vi "FIFO IN.vi"(8 "error in (no error)":errorcluster, 11 "Engine Run-Time Data Cluster In":T1 {"Compiled Data"."Corruption Info DUT_Network"."Frame Infos Array"."CRC Index" min=-7 max=7; "Compiled Data"."Corruption Info DUT_Network"."Frame Infos Array"."DLC Length  Corruption Index" min=-8 max=8; "Compiled Data"."Corruption Info Network_DUT"."Frame Infos Array"."CRC Index" min=-7 max=7; "Compiled Data"."Corruption Info Network_DUT"."Frame Infos Array"."DLC Length  Corruption Index" min=-8 max=8; "Specified Channel Ref List Out" format="%.0x"; "Specified Channel Ref List In" format="%.0x"}) -> (0 "error out":errorcluster, 3 "Engine Run-Time Data Cluster Out":T1 {"Compiled Data"."Corruption Info DUT_Network"."Frame Infos Array"."CRC Index" min=-7 max=7; "Compiled Data"."Corruption Info DUT_Network"."Frame Infos Array"."DLC Length  Corruption Index" min=-8 max=8; "Compiled Data"."Corruption Info Network_DUT"."Frame Infos Array"."CRC Index" min=-7 max=7; "Compiled Data"."Corruption Info Network_DUT"."Frame Infos Array"."DLC Length  Corruption Index" min=-8 max=8; "Specified Channel Ref List Out" format="%.0x"; "Specified Channel Ref List In" format="%.0x"})   [LabVIEW 2018, in "CAN Gateway Engine.lvlib"]
uses:
  CAN Gateway Engine.lvlib
  Shared/CTLs/Runtime engine Data.ctl
  <vilib>/NI Veristand/Custom Device API/Custom Device Engine Event Ref.ctl
  <vilib>/NI Veristand/Custom Device API/Custom Device Item Ref.ctl
  Shared/CTLs/Compiled Data.ctl
  Shared/CTLs/Corruption Info.ctl
  Shared/CTLs/Frame.ctl
  Shared/CTLs/Signal_Data_Trigger.ctl
  <vilib>/NI Veristand/Custom Device API/Custom Device API.lvlib
  Shared/CAN Gateway Shared.lvlib
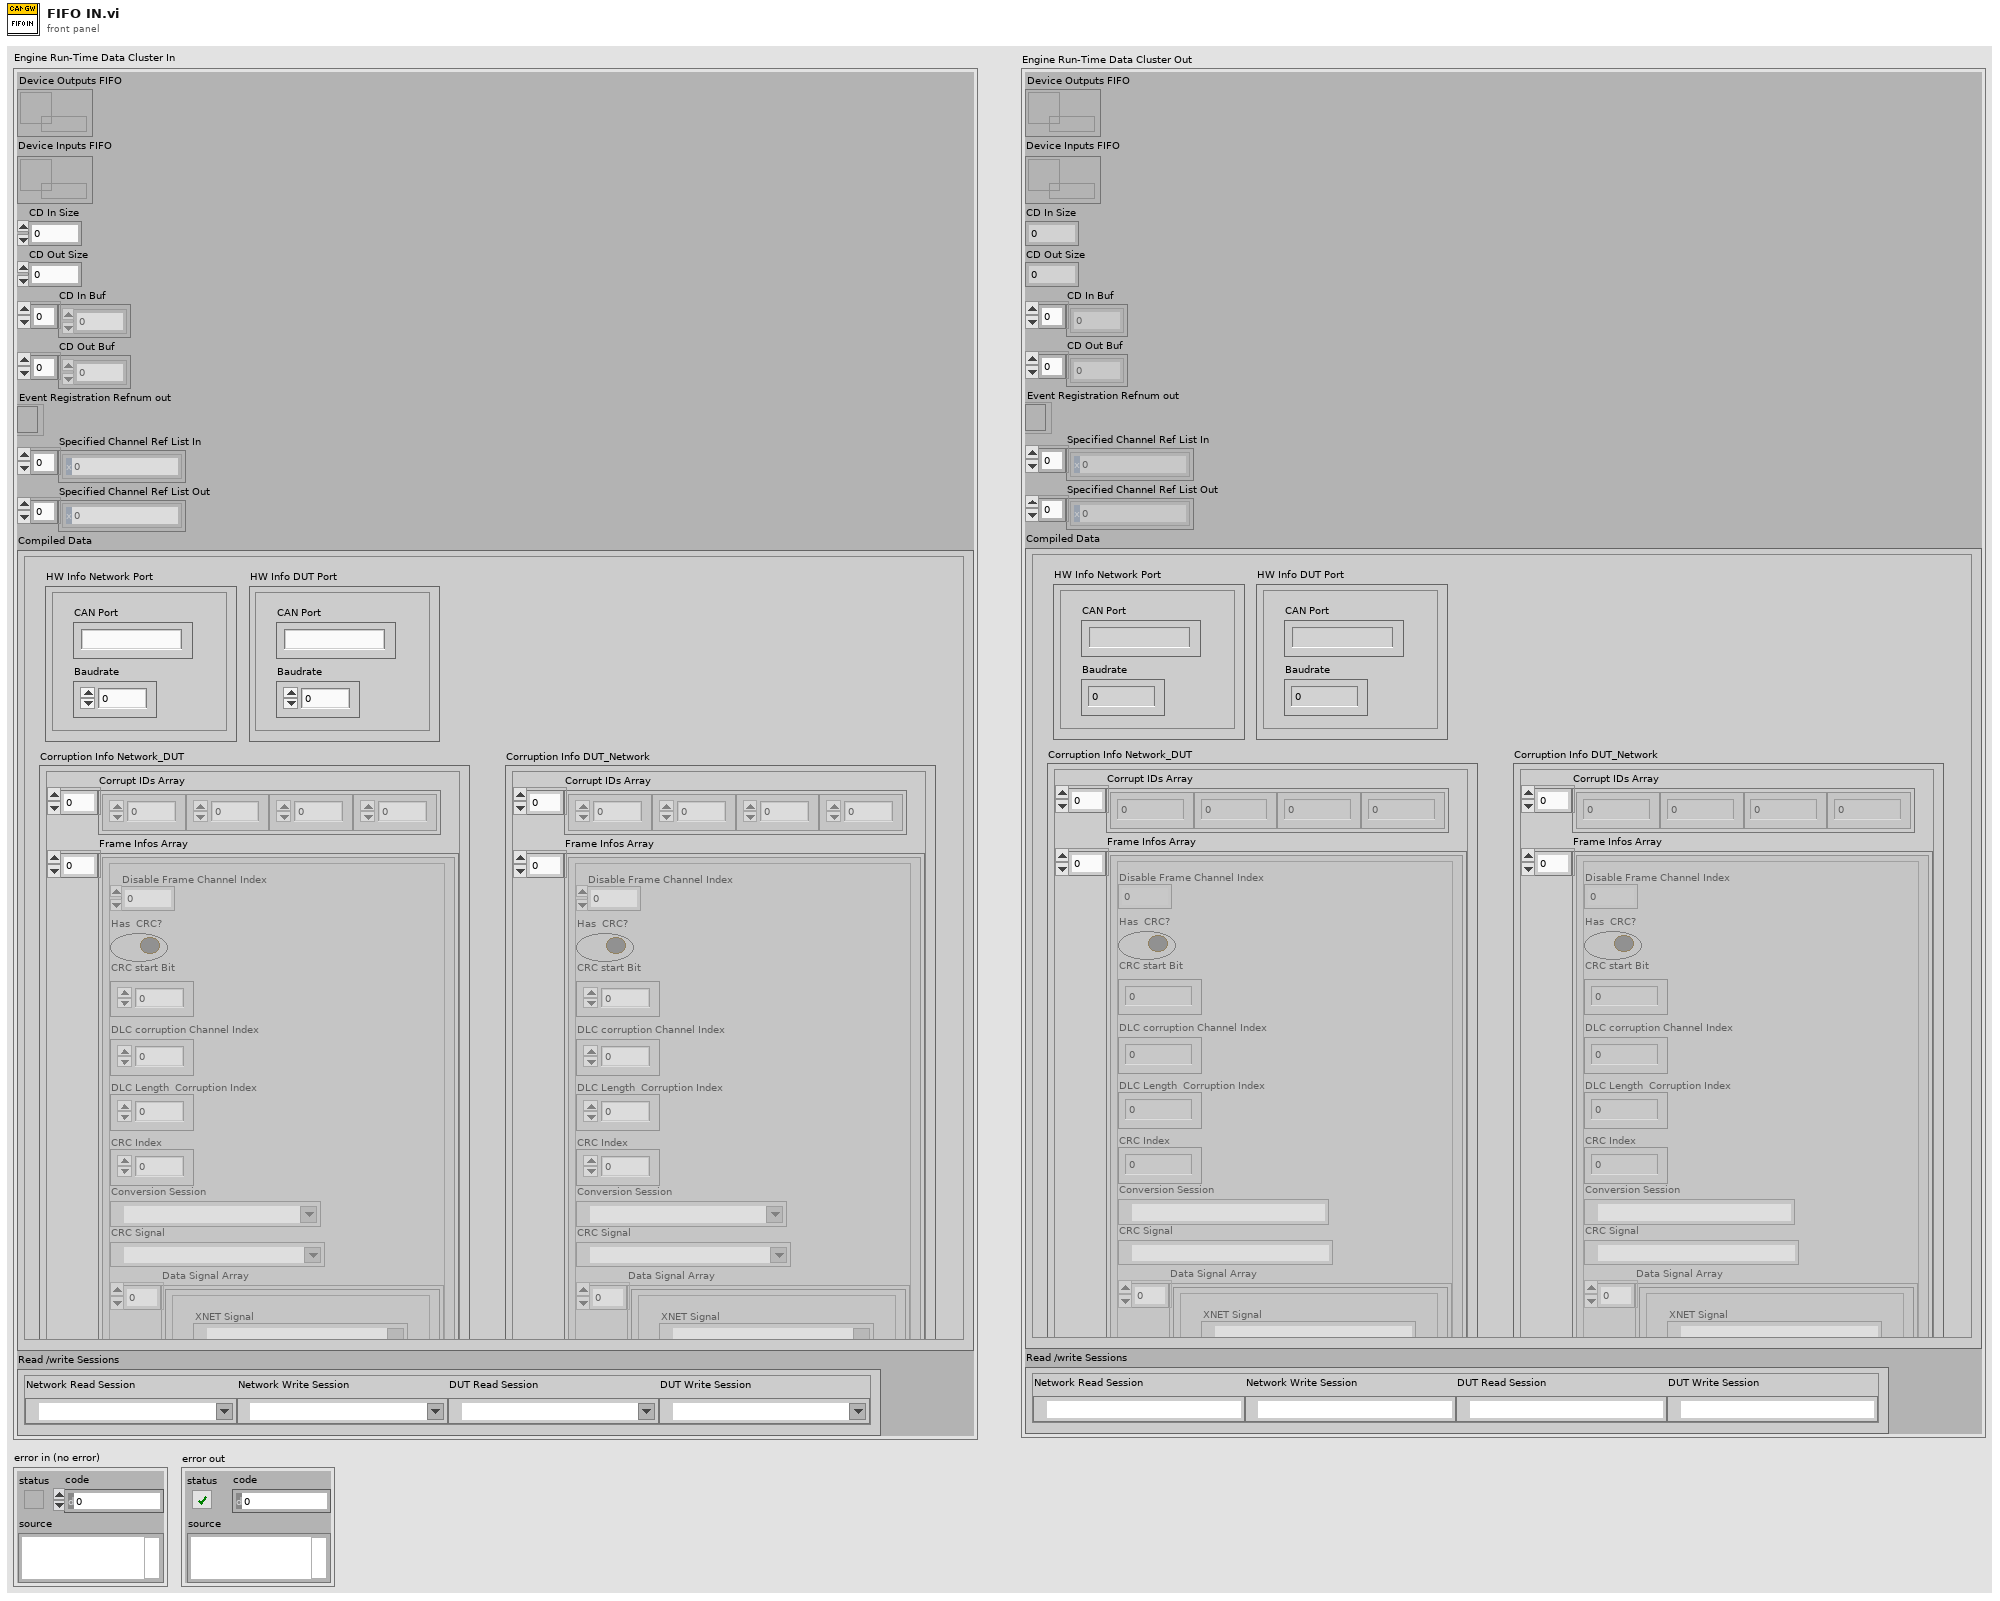
[diagram p1: front panel]
types:
  T1 = typedef "CAN Gateway Engine.lvlib/Runtime engine Data.ctl" = cluster{"Device Outputs FIFO":refnum<k33>, "Device Inputs FIFO":refnum<k33>, "CD In Size":i32, "CD Out Size":i32, "CD In Buf":dbl[], "CD Out Buf":dbl[], "Event Registration Refnum out":T2, "Specified Channel Ref List In":T3[], "Specified Channel Ref List Out":T3[], "Compiled Data":T4, "Read /write Sessions":cluster{"Network Read Session":refnum<k21>, "Network Write Session":refnum<k21>, "DUT Read Session":refnum<k21>, "DUT Write Session":refnum<k21>}}
  T2 = typedef "Custom Device API.lvlib/Custom Device Engine Event Ref.ctl" = refnum<event-registration>
  T3 = typedef "Custom Device API.lvlib/Custom Device Item Ref.ctl" = u64
  T4 = typedef "CAN Gateway Shared.lvlib/Compiled Data.ctl" = cluster{"HW Info Network Port":cluster{"CAN Port":string, "Baudrate":u64}, "HW Info DUT Port":cluster{"CAN Port":string, "Baudrate":u64}, "Corruption Info Network_DUT":T5, "Corruption Info DUT_Network":T5}
  T5 = typedef "CAN Gateway Shared.lvlib/Corruption Info.ctl" = cluster{"Corrupt IDs Array":u32[], "Frame Infos Array":T6[]}
  T6 = typedef "CAN Gateway Shared.lvlib/Frame.ctl" = cluster{"Disable Frame Channel Index":i32, "Has  CRC?":bool, "CRC start Bit":u32, "DLC corruption Channel Index":i32, "DLC Length  Corruption Index":i32, "CRC Index":i32, "Conversion Session":refnum<k21>, "CRC Signal":refnum<k21>, "Data Signal Array":T7[]}
  T7 = typedef "CAN Gateway Shared.lvlib/Signal_Data_Trigger.ctl" = cluster{"XNET Signal":refnum<k21>, "Data Idx":u32, "Trigger Idx":u32}
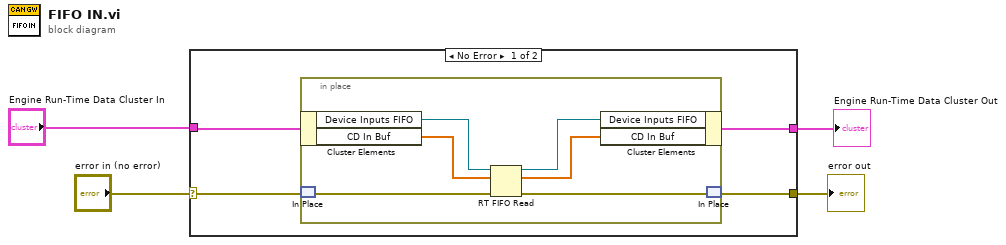
[diagram p0: block diagram]
diagram:
  n1 = case shown="No Error" "error in (no error)" {
    selector: "error in (no error)" -> [w6 w16]
    tunnel: [w5 w16] -> w3
    tunnel: "Engine Run-Time Data Cluster In" -> [w8 w15]
    tunnel: [w7 w15] -> w1
    frame No Error {
      n2 = in-place {
        n3 = in-place-cluster #1(w8) -> ("Device Inputs FIFO"=w14:refnum<k33>, "CD In Buf"=w13:dbl[])
        n4 = in-place-match #2(w6) -> (w10:errorcluster)
        n5 = RT FIFO Read(0:w14, 1:w13, 3:w10) -> (8:w12:refnum<k33>, 9:w11:dbl[], 11:w9:errorcluster)  [unwired: 1 in, 2 out]
        n6 = in-place-cluster #1("Device Inputs FIFO"=w12, "CD In Buf"=w11) -> (w7:T1)
        n7 = in-place-match #2(w9) -> (w5:errorcluster)
      }
    }
    frame Error {
    }
  }
  "error out" <- w3
  "Engine Run-Time Data Cluster Out" <- w1
